vi "WriteData.vi"(8 "error in":errorcluster, 9 "Data(0~8Byte)":u8[](array[numeric]), 10 "ID":u32, 11 "VISA Refnum in":refnum<visa-resource-name>) -> (0 "error out":errorcluster, 3 "VISA Refnum out":refnum<visa-resource-name>)   [LabVIEW 2019, in "CubeMarsBLDClib.lvlib"]
uses:
  CubeMarsBLDClib.lvlib
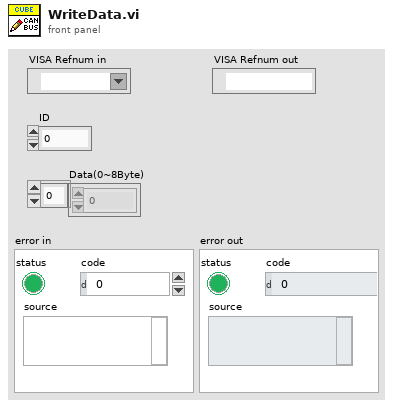
[diagram p1: front panel]
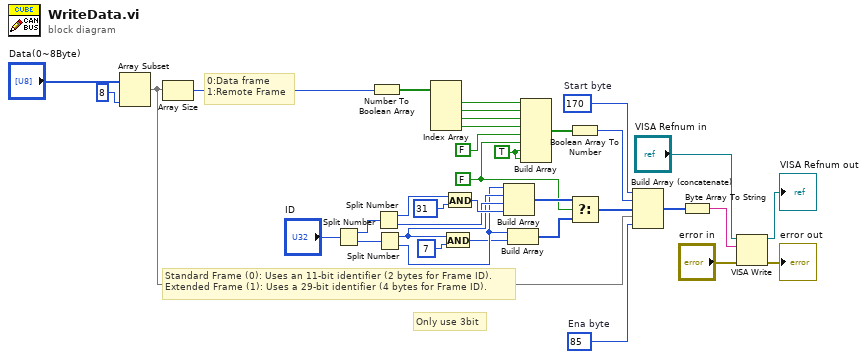
[diagram p0: block diagram]
diagram:
  w36 = u8 85  # Ena byte
  w16 = TRUE ("element")
  w25 = FALSE
  w18 = u8 170  # Start byte
  # "Only use 3bit"
  # "Standard Frame (0): Uses an 11-bit identifier (2 bytes for Frame ID).\nExtended Frame (1): Uses a 29-bit identifier (4 bytes for Frame ID)."
  # "0:Data frame\n1:Remote Frame"
  n1 = Array Subset(array="Data(0~8Byte)", length=8) -> (w5:u8[])  [unwired: 1 in]
  n2 = Array Size(array=w5) -> (size(s)=w9:i32)
  n3 = Split Number(x="ID") -> (hi(x)=w21:u16, lo(x)=w22:u16)
  n4 = Number To Boolean Array(number=w9) -> (Boolean array=w10:bool[])
  n5 = Split Number(x=w21) -> (hi(x)=w30:u8, lo(x)=w29:u8)
  n6 = Split Number(x=w22) -> (hi(x)=w28:u8, lo(x)=w27:u8)
  n7 = Index Array(array=w10) -> (element #1=w11:bool, element #2=w12:bool, element #3=w13:bool, element #4=w14:bool)  [unwired: 4 in]
  n8 = And(x=w28, y=u8 7) -> (x .and. y?=w24:u8)
  n9 = And(x=w30, y=u8 31) -> (x .and. y?=w32:u8)
  n10 = Build Array(w27, w28, w29, w32) -> (w33:u8[])
  n11 = Build Array(w27, w24) -> (w26:u8[])
  n12 = Build Array(w11, w12, w13, w14, FALSE, w25, w16, w16) -> (w17:bool[])
  n13 = Boolean Array To Number(Boolean array=w17) -> (number=w19:u8)
  n14 = Select(t=w33, s=w25, f=w26) -> (s? t:f=w34:u8[])
  n15 = Build Array (concatenate)(w18, w19, w34, w5, w36) -> (w35:u8[])
  n16 = Byte Array To String(unsigned byte array=w35) -> (string=w6:string)
  n17 = VISA Write(VISA resource name="VISA Refnum in", write buffer=w6, error in (no error)="error in") -> (VISA resource name out=→"VISA Refnum out":refnum<visa-resource-name>, error out=→"error out":errorcluster)  [unwired: 1 out]
